vi "testDriveLoop.vi"() -> ()   [LabVIEW 2018]
uses:
  <vilib>/Platform/TimedLoop/XDataNode/timing_clust.ctl
  <vilib>/Platform/TimedLoop/XDataNode/nitl_modes.ctl
  <vilib>/Platform/TimedLoop/XDataNode/wakeup.ctl
  <vilib>/Rock Robotics/WPI/ThirdParty/Phoenix-LabVIEW/Motor Controller/Controls/CTRE_Phoenix_MotorControl_ControlMode.ctl
  driveShifterEnum.ctl
  <vilib>/platform/TimedLoop/XDataNode/XDataNode.xnode
  <vilib>/Platform/TimedLoop/XDataNode/XDNodeRunTimeDep.lvlib
panel:
  out "Iteration Duration":i64(graph)
  in  "Quickturn_Sens_Low":dbl=1.0
  in  "Quickturn_Sens_High":dbl=0.6 format="%#_13g"
  in  "speed limit":dbl=1.0
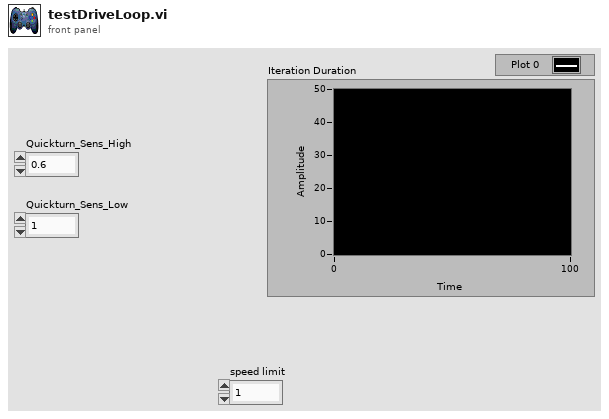
[diagram p1: front panel]
types:
  T1 = typedef "XDNodeRunTimeDep.lvlib/timing_clust.ctl" = cluster{"Expected End [f-1]":u64, "Actual End [f-1]":u64, "Finished Late? [f-1]":bool, "Expected End [i-1]":u64, "Actual End [i-1]":u64, "Finished Late? [i-1]":bool, "Expected Start [i]":u64, "Actual Start [i]":u64, "Expected Start [f]":u64, "Actual Start [f]":u64, "Source Name":string, "Structure Name":string, "Period":i64, "Deadline":i64, "Offset":i64, "Start":i64, "Priority":i32, "Timeout":i32, "Mode":T2, "Wakeup Reason":T3, "Error":errorcluster, "Source Type":string, "Secondary Source Type":string, "Global End Time":u64, "Global Start Time":u64, "Frame Duration":u64, "Iteration Duration":u64, "Assigned CPU":i32, "I/O Scan Engine Mode":u32}
  T2 = typedef "XDNodeRunTimeDep.lvlib/nitl_modes.ctl" = enum32{"No Change", "Process missed periods, maintain original phase", "Discard missed periods, maintain original phase", "Process missed periods, ignore original phase", "Discard missed periods, ignore original phase"}
  T3 = typedef "XDNodeRunTimeDep.lvlib/wakeup.ctl" = enum32{"Normal", "Aborted", "Asynchronous wakeup", "Timing source error", "Timed loop error", "Timeout"}
  T4 = typedef "WPI_MotorControlDeviceRef.ctl" = cluster{"DeviceStatus":errorcluster, "Type":T5, "PWM":cluster{"PWM Channel":T6, "DeadBand":T7}, "CAN":cluster{"Device Number":u8, "SetOutput VI Ref":variant, "GetOutput VI Ref":variant, "Enable VI Ref":variant, "Disable VI Ref":variant, "Data":variant}, "Invert":bool, "DIO PWM":cluster{"PWM \"Enable\" Channel":T6, "DIOChannel":T8, "PWM Rate":dbl}}
  T5 = typedef "WPI_MotorControlType.ctl" = enum16{"PWM", "CAN", "DIO PWM"}
  T6 = typedef "FPGA_DIOPWMChannel.ctl" = enum8{"PWM 0", "PWM 1", "PWM 2", "PWM 3", "PWM 4", "PWM 5", "PWM 6", "PWM 7", "PWM 8", "PWM 9", "PWM MXP 0", "PWM MXP 1", "PWM MXP 2", "PWM MXP 3", "PWM MXP 4", "PWM MXP 5", "PWM MXP 6", "PWM MXP 7", "PWM MXP 8", "PWM MXP 9", "Invalid"}
  T7 = typedef "WPI_PWMDeadband.ctl" = cluster{"Name":string, "maxPositivePwm":i32, "minPositivePwm":i32, "centerPwm":i32, "maxNegativePwm":i32, "minNegativePwm":i32, "angularRange":u16}
  T8 = typedef "FPGA_DIOChannel.ctl" = enum8{"DIO 0", "DIO 1", "DIO 2", "DIO 3", "DIO 4", "DIO 5", "DIO 6", "DIO 7", "DIO 8", "DIO 9", "DIO MXP 0", "DIO MXP 1", "DIO MXP 2", "DIO MXP 3", "DIO MXP 4", "DIO MXP 5", "DIO MXP 6", "DIO MXP 7", "DIO MXP 8", "DIO MXP 9", "DIO MXP 10", "DIO MXP 11", "DIO MXP 12", "DIO MXP 13", "DIO MXP 14", "DIO MXP 15", "SPI Port CS1", "SPI Port CS2", "SPI Port CS3", "SPI Port MISO", "SPI Port MOSI", "Invalid"}
  T9 = typedef "driveShifterEnum.ctl" = enum16{"Low", "High"}
  T10 = cluster{"Quickturn_Sens_High":dbl, "Quickturn_Sens_Low":dbl}
  T11 = typedef "CTRE_Phoenix_MotorControl_ControlMode.ctl" = u16
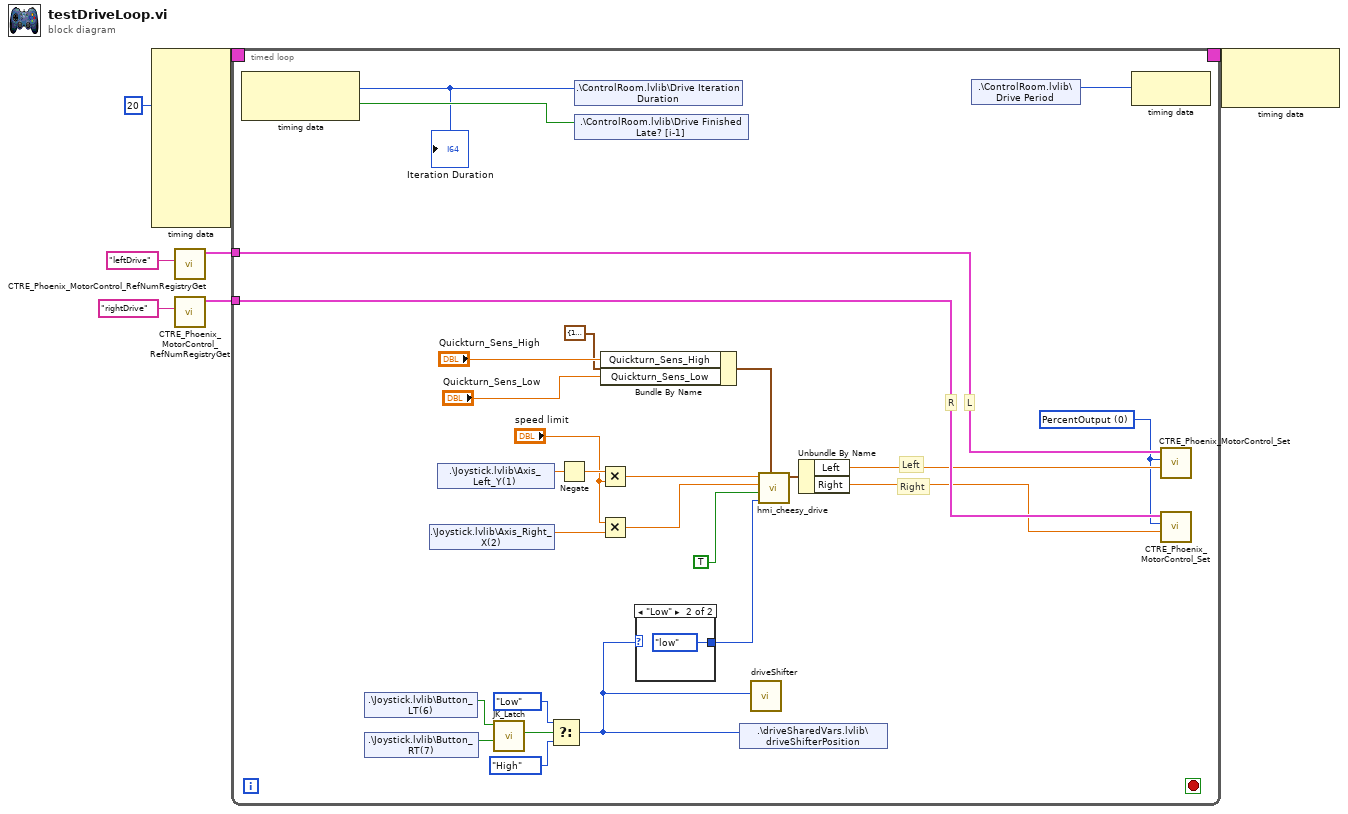
[diagram p0: block diagram]
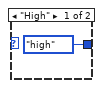
[diagram p2: hidden frame]
diagram:
  n1 = node-c288(20 ("Priority")) -> (w7:T1)  [unwired: 9 in]
  n2 = call <vilib>:"CTRE_Phoenix_MotorControl_RefNumRegistryGet.vi"("refnum name"="leftDrive") -> ("PhoenixMotorControlDevRef"=w3:T4)  [unwired: 9 in, 1 out]
  n3 = call <vilib>:"CTRE_Phoenix_MotorControl_RefNumRegistryGet.vi"("refnum name"="rightDrive") -> ("PhoenixMotorControlDevRef"=w2:T4)  [unwired: 9 in, 1 out]
  n4 = timed-loop {
    timing: w7 -> [_]
    timing-out: [_] -> w6
    tunnel: w3 -> [w34]
    tunnel: w2 -> [w33]
    stop <- _ stop-if-true
    w26 = T11 0 items=["PercentOutput"=0, "Position"=1, "Velocity"=2, "Current"=3, "Follower"=5, "MotionProfile"=6, "MotionMagic"=7, "MotionProfileArc"=10, "Disabled"=15] ("Control Mode")
    # "Right"
    # "Left"
    # "L"
    # "R"
    n5 = node-c288() -> (w27:i64, w28:bool)  [unwired: 1 in]
    "Iteration Duration" <- w27
    n6 = shared-variable ".\\Joystick.lvlib\\Button_LT(6)"() -> (w8:bool)  [unwired: 1 in, 1 out]
    n7 = shared-variable ".\\Joystick.lvlib\\Button_RT(7)"() -> (w9:bool)  [unwired: 1 in, 1 out]
    n8 = shared-variable ".\\Joystick.lvlib\\Axis_Right_X(2)"() -> (w24:dbl)  [unwired: 1 in, 1 out]
    n9 = shared-variable ".\\Joystick.lvlib\\Axis_Left_Y(1)"() -> (w25:dbl)  [unwired: 1 in, 1 out]
    n10 = call <userlib>:"JK_Latch.vi"("Reset"=w9, "Set"=w8) -> ("Q"=w10:bool)  [unwired: 5 in]
    n11 = Select(t=driveShifterEnum."Low", s=w10, f=driveShifterEnum."High") -> (s? t:f=w32:T9)
    n12 = Negate(x=w25) -> (-x=w23:dbl)
    n13 = shared-variable ".\\ControlRoom.lvlib\\Drive Iteration Duration"(w27) -> ()  [unwired: 1 in, 1 out]
    n14 = shared-variable ".\\ControlRoom.lvlib\\Drive Finished Late? [i-1]"(w28) -> ()  [unwired: 1 in, 1 out]
    n15 = Multiply(x=w23, y="speed limit") -> (x*y=w19:dbl)
    n16 = Multiply(x="speed limit", y=w24) -> (x*y=w20:dbl)
    n17 = Bundle By Name(cluster=T10 {"Quickturn_Sens_High"=1.0, "Quickturn_Sens_Low"=1.0} ("Sens Values"), "Quickturn_Sens_High"="Quickturn_Sens_High", "Quickturn_Sens_Low"="Quickturn_Sens_Low") -> (w16:T10)
    n18 = case shown="\"Low\"" w32 {
      tunnel: [enum16{"low", "high"}."high" ("gear shift state") enum16{"low", "high"}."low" ("gear shift state")] -> w14
      frame "High" {
      }
      frame "Low" {
      }
    }
    n19 = shared-variable ".\\driveSharedVars.lvlib\\driveShifterPosition"(w32) -> ()  [unwired: 1 in, 1 out]
    n20 = call "driveShifter.vi"(10:w32) -> ()  [unwired: 11 in]
    n21 = call <userlib>:"hmi_cheesy_drive.vi"("Sens Values"=w16, "gear shift state"=w14, "Quick Turn"=TRUE, "Wheel"=w20, "Throttle"=w19) -> ("Drive Data"=w22:cluster{"Left":dbl, "Right":dbl})  [unwired: 6 in]
    n22 = Unbundle By Name(w22) -> ("Left"=w30:dbl, "Right"=w31:dbl)
    n23 = shared-variable ".\\ControlRoom.lvlib\\Drive Period"() -> (w29:i64)  [unwired: 1 in, 1 out]
    n24 = node-c288(w29) -> ()  [unwired: 1 out]
    n25 = call <vilib>:"CTRE_Phoenix_MotorControl_Set.vi"("Output"=w30, "Control Mode"=w26, "PhoenixMotorControlDevRef"=w34) -> ()  [unwired: 7 in, 2 out]
    n26 = call <vilib>:"CTRE_Phoenix_MotorControl_Set.vi"("Output"=w31, "Control Mode"=w26, "PhoenixMotorControlDevRef"=w33) -> ()  [unwired: 7 in, 2 out]
  }
  n27 = node-c288(w6) -> ()  [unwired: 2 out]
